vi "SimpleFileWrite.vi"() -> ()   [LabVIEW 2017]
panel:
  out "TDMS path":path
  in  "Log File Name":string="FileWriteTest1"
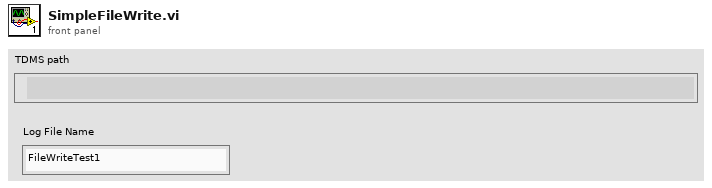
[diagram p1: front panel]
types:
  T1 = enum16{"open", "open or create", "create or replace", "create", "open (read-only)"}
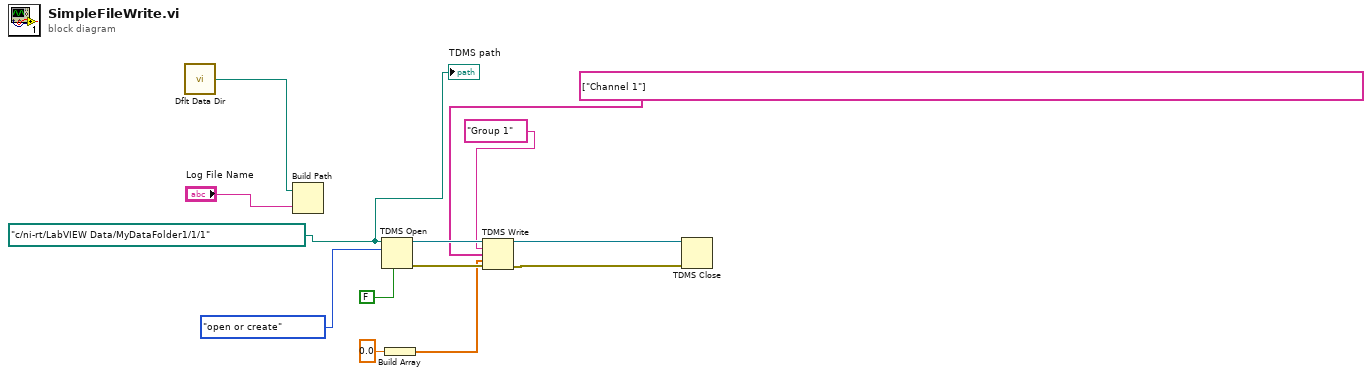
[diagram p0: block diagram]
diagram:
  w1 = path "c:/ni-rt/LabVIEW Data/MyDataFolder1/1/1" ("appended path")
  n1 = call <vilib>:"Dflt Data Dir.vi"() -> ("App:Default Data Directory"=w2:path)
  n2 = Build Path(base path=w2, name or relative path="Log File Name") -> ()  [unwired: 1 out]
  n3 = TDMS Open(6:FALSE ("disable buffering (T)"), 10:T1."open or create" ("operation"), 11:w1) -> (0:w9:errorcluster, 3:w11:refnum<k34>)  [unwired: 4 in]
  n4 = Build Array(0.0 ("element")) -> (w5:dbl[])
  n5 = TDMS Write(0:w11, 5:"Group 1" ("group name in (Untitled)"), 7:string[] ["Channel 1"] ("channel name(s) in (Untitled)"), 9:w5, 11:w9) -> (4:w10:refnum<k34>, 15:w8:errorcluster)  [unwired: 1 in, 2 out]
  n6 = TDMS Close(8:w8, 11:w10) -> ()  [unwired: 2 out]
  "TDMS path" <- w1
